vi "Run_Expand_Constraints_decomposition.vi"() -> ()   [LabVIEW 2019]
uses:
  <vilib>/Utility/file.llb/Read Delimited Spreadsheet (DBL).vi
panel:
  out "output cluster":T1
  in  "Lq":i32=15
  out "OmegaChain":dbl[](array[numeric])
  out "beta":dbl[](array[numeric])
  out "gamma":dbl
  out "weight":dbl
  in  "w0":dbl=100000.0
  out "Nc":i32
  out "one constraint":dbl[](array[numeric])
  out "size(s)":i32[](array[numeric])
  out "all constraints":dbl[][](array[numeric])
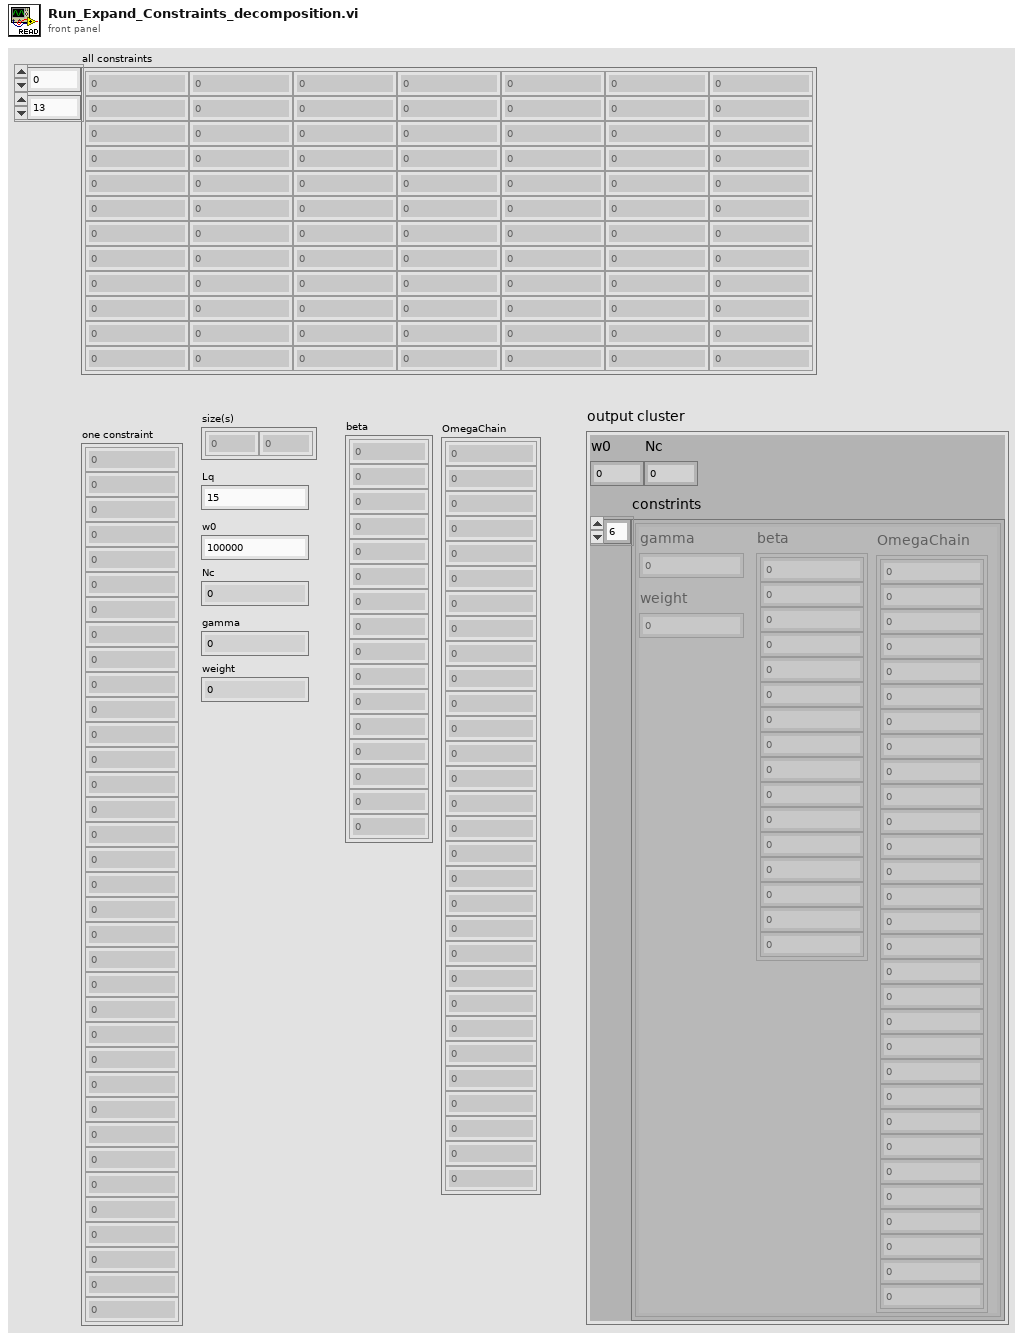
[diagram p1: front panel]
types:
  T1 = cluster{"w0":dbl, "constrints":cluster{"beta":dbl[], "gamma":dbl, "OmegaChain":dbl[], "weight":dbl}[], "Nc":i32}
  T2 = cluster{"beta":dbl[], "gamma":dbl, "OmegaChain":dbl[], "weight":dbl}
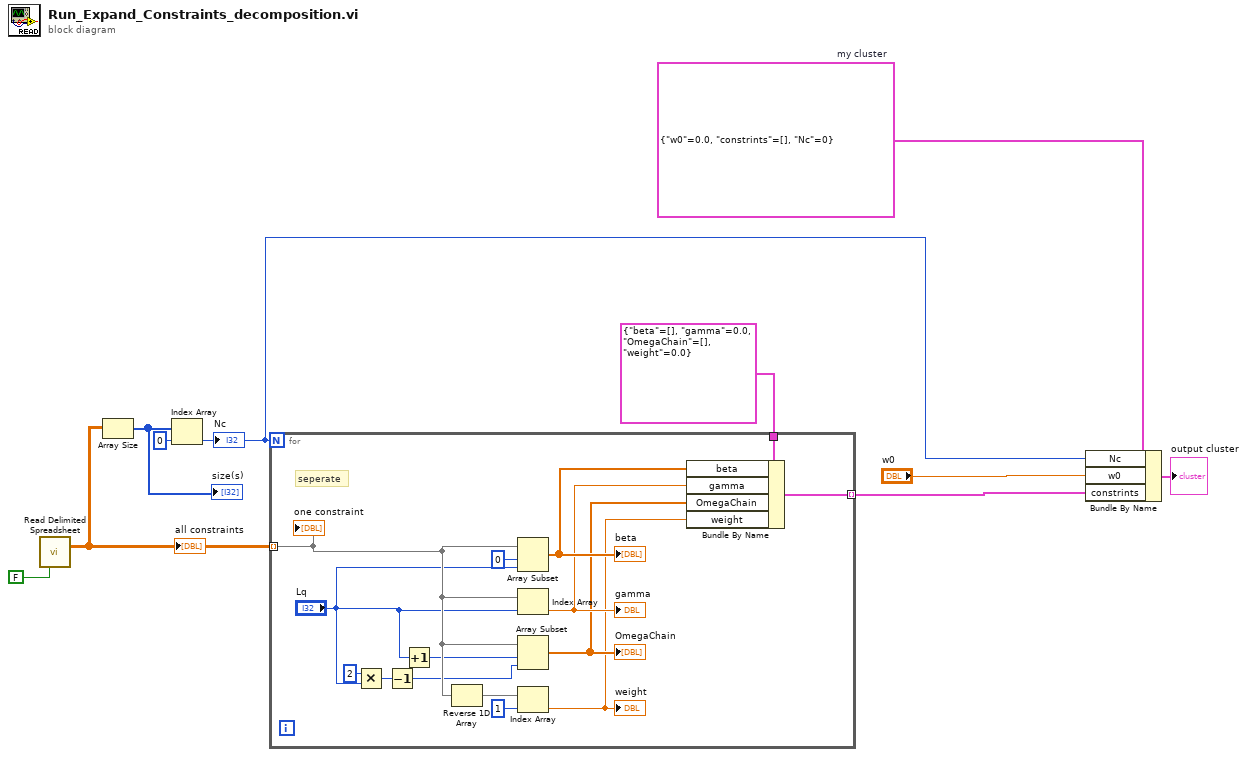
[diagram p0: block diagram]
diagram:
  w5 = T1 {"w0"=0.0, "constrints"=[], "Nc"=0}  # my cluster
  n1 = call-poly <vilib>:"Read Delimited Spreadsheet.vi"("transpose? (F)"=FALSE) -> ("all rows"=w7:dbl[][])  [unwired: 9 in, 5 out]
  "all constraints" <- w7
  n2 = Array Size(array=w7) -> (size(s)=w9:i32[])
  "size(s)" <- w9
  n3 = Index Array(array=w9, index=0) -> (element=w3:i32)
  "Nc" <- w3
  n4 = for {
    N: w3 -> [_]
    tunnel: w7 -> [w25] mode=indexing
    tunnel: [w11] -> w4 mode=indexing
    tunnel: T2 {"beta"=[], "gamma"=0.0, "OmegaChain"=[], "weight"=0.0} -> [w16]
    # "seperate"
    n5 = Multiply(x=2, y="Lq") -> (x*y=w20:i32)
    n6 = Decrement(x=w20) -> (x-1=w19:i32)
    n7 = Increment(x="Lq") -> (x+1=w22:i32)
    n8 = Reverse 1D Array(array=w25) -> (reversed array=w18:dbl[])
    n9 = Array Subset(array=w25, index=0, length="Lq") -> (w15:dbl[])
    "beta" <- w15
    n10 = Index Array(array=w25, index="Lq") -> (element=w14:dbl)
    "gamma" <- w14
    n11 = Array Subset(array=w25, index=w22, length=w19) -> (w13:dbl[])
    "OmegaChain" <- w13
    n12 = Index Array(array=w18, index=1) -> (element=w12:dbl)
    "weight" <- w12
    n13 = Bundle By Name(cluster=w16, "beta"=w15, "gamma"=w14, "OmegaChain"=w13, "weight"=w12) -> (w11:T2)
    "one constraint" <- w25
  }
  n14 = Bundle By Name(cluster=w5, "Nc"=w3, "w0"="w0", "constrints"=w4) -> (→"output cluster":T1)
